vi "Light Config Const.vi"() -> (2 "Light Config":T1={"Desk Left"="192.168.42.98", "Desk Right"="192.168.42.135", "Printer"="192.168.42.101"})   [LabVIEW 2022 SP3, in "TouchControl.lvlib"]
uses:
  TouchControl.lvlib
  Light Config.ctl
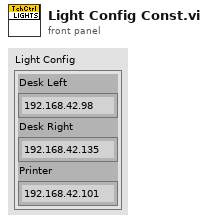
[diagram p1: front panel]
types:
  T1 = typedef "TouchControl.lvlib/Light Config.ctl" = cluster{"Desk Left":string, "Desk Right":string, "Printer":string}
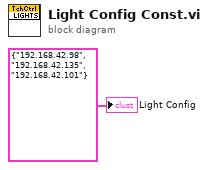
[diagram p0: block diagram]
diagram:
  "Light Config" <- T1 {"Desk Left"="192.168.42.98", "Desk Right"="192.168.42.135", "Printer"="192.168.42.101"} ("Light Config")
